vi "GDSAPI_ChangeInheritance.vi"(8 "error in (no error)":errorcluster, 10 "NewParentClassPath(*.lvclass), leave empty to make it a base class":path, 11 "ClassPath(*.lvclass)":path) -> (0 "error out":errorcluster, 3 "ClassPathOut(*.lvclass)":path)   [LabVIEW 2020]
doc: "This VI changes the inheritance of classes"
uses:
  <resource>/Framework/Providers/Open_GDS/ClassProviders/Provider_LvNativeClass/ClassWriterNative_class/ClassWriterNative.lvclass
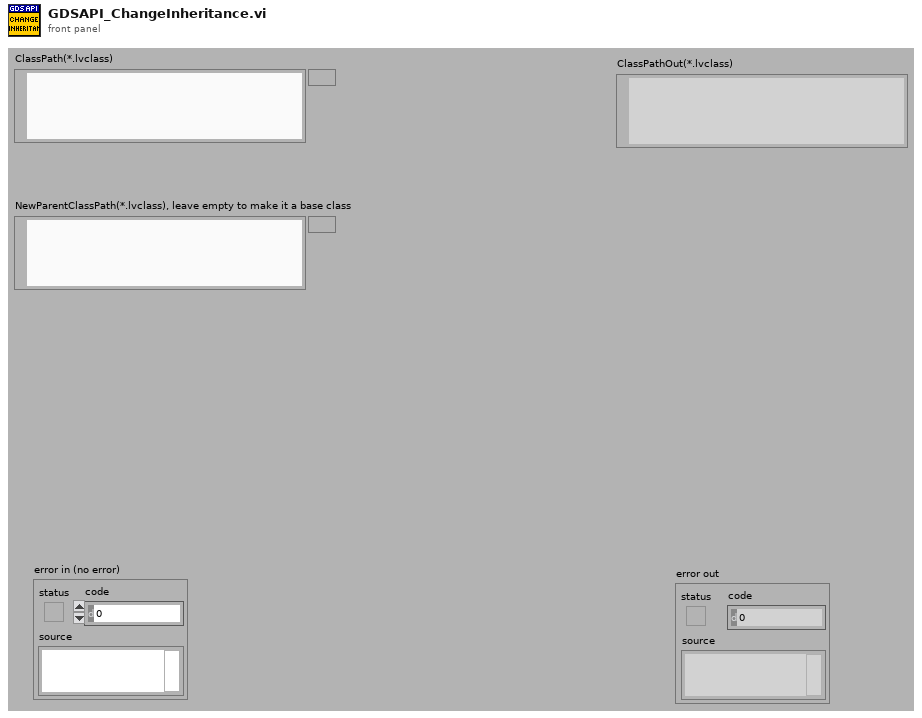
[diagram p1: front panel]
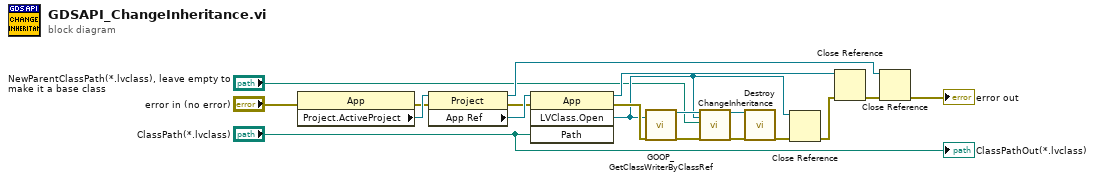
[diagram p0: block diagram]
diagram:
  n1 = property class="App"(error in="error in (no error)") -> (error out=w14:errorcluster, "Project.ActiveProject"=w17:refnum<vi>)  [unwired: 1 in, 1 out]
  n2 = property class="Project"(reference=w17, error in=w14) -> (reference out=w9:refnum<vi>, error out=w15:errorcluster, "App Ref"=w16:refnum<vi>)
  n3 = invoke class="App" method="LVClass.Open"(reference=w16, error in=w15, "Path"="ClassPath(*.lvclass)") -> (reference out=w11:refnum<vi>, error out=w18:errorcluster, "LVClass.Open"=w2:refnum<vi>)  [unwired: 1 in, 1 out]
  n4 = call <resource>:"GOOP_GetClassWriterByClassRef.vi"("LVClassLibrary Refnum"=w2, "error in (no error)"=w18) -> ("ClassWriterNative.lvclass"=w6:refnum<class "ClassWriterNative.lvclass">, "error out"=w3:errorcluster)  [unwired: 16 in]
  n5 = call-dynamic "ChangeInheritance.vi"("ClassWriterGOOP300 in"=w6, "LvClass"=w2, "NewBaseClass(Empty=ConvertClassToBaseClass)"="NewParentClassPath(*.lvclass), leave empty to make it a base class", "error in (no error)"=w3) -> ("ClassWriterGOOP300 out"=w5:refnum<class "ClassWriterNative.lvclass">, "error out"=w4:errorcluster)  [unwired: 14 in]
  n6 = call-dynamic "Destroy.vi"("ClassWriterNative"=w5, "error in (no error)"=w4) -> ("error out"=w19:errorcluster)  [unwired: 17 in]
  n7 = Close Reference(reference=w2, error in (no error)=w19) -> (error out=w12:errorcluster)
  n8 = Close Reference(reference=w11, error in (no error)=w12) -> (error out=w10:errorcluster)
  n9 = Close Reference(reference=w9, error in (no error)=w10) -> (error out=→"error out":errorcluster)
  "ClassPathOut(*.lvclass)" <- "ClassPath(*.lvclass)"
